vi "Calibrate sensor main.vi"() -> ()   [LabVIEW 2024]
doc: "Calibration VI"
uses:
  controls/Units.ctl
  <vilib>/Utility/miscctls.llb/LVPointTypeDef.ctl
  controls/Cal Sensor Enum.ctl
  controls/GlobalData.vi
  <userlib>/_OpenG.lib/lvdata/lvdata.llb/openg_variant.lvlib
panel:
  in  "Units Settings":T1={"Pressure"=enum."Pa", "Temperature"=enum."F", "Salinity"=enum."ppt", "Weight"=enum."ib"}
  in  "Cancel Button":bool
  in  "Weight":T2={"W C (Y-Intercept)"=0.0, "W M (Gradient)"=100.0, "Zero Weight"=FALSE, "Weight %s"=22.86994789, "W Current (mA)"=0.0, "W Save Calibration"=FALSE} {"W Current (mA)" format="%#_12g"; "Weight %s" scale=0.0..220.0}
  in  "Salinity":T3={"S C (Y-Intercept)"=0.0, "S M (Gradient)"=100.0, "Zero Salinity"=FALSE, "Salinity %s"=0.0, "S Current (mA)"=0.0, "S Save Calibration"=FALSE} {"S Current (mA)" format="%#_12g"; "Salinity %s" scale=0.0..100000.0}
  in  "Temperature":T4={"T C (Y-Intercept)"=0.0, "T M (Gradient)"=100.0, "Zero Temperature"=FALSE, "Temperature %s"=0.0, "T Current (mA)"=0.0, "T Save Calibration"=FALSE} {"T Current (mA)" format="%#_12g"; "Temperature %s" scale=0.0..100.0}
  in  "Pressure":T5={"P C (Y-Intercept)"=0.0, "P M (Gradient)"=3.0, "Zero pressure"=FALSE, "Pressure %s"=36.73931247994955, "P Current (mA)"=36.73931247994955, "P Save Calibration"=FALSE} {"P Current (mA)" format="%#_12g"; "Pressure %s" scale=0.0..60.0}
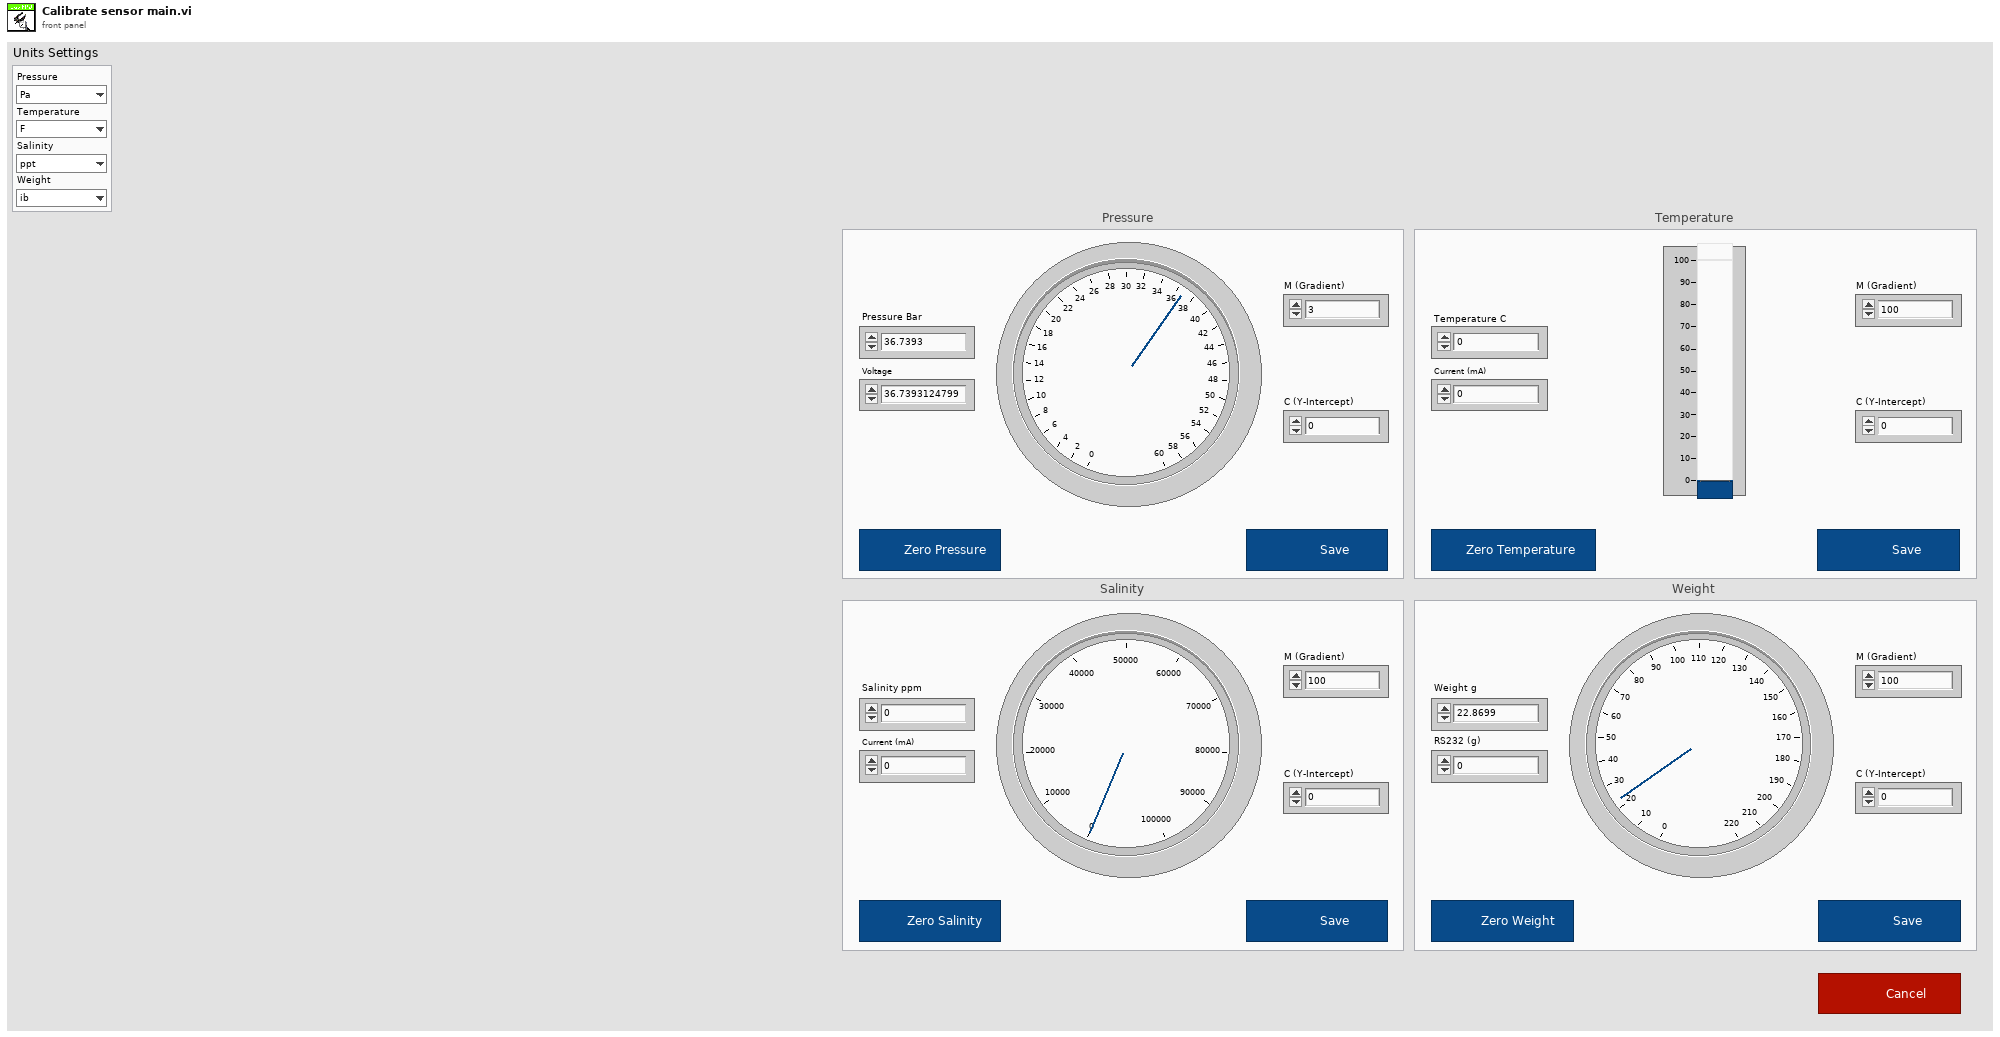
[diagram p1: front panel]
types:
  T1 = typedef "Units.ctl" = cluster{"Pressure":enum16{"PSI", "Bar", "atm", "Pa"}, "Temperature":enum16{"C", "K", "F"}, "Salinity":enum16{"ppm", "ppt", "PSU"}, "Weight":enum16{"Kg", "g", "oz", "ib"}}
  T2 = cluster{"W C (Y-Intercept)":dbl, "W M (Gradient)":dbl, "Zero Weight":bool, "Weight %s":dbl, "W Current (mA)":dbl, "W Save Calibration":bool}
  T3 = cluster{"S C (Y-Intercept)":dbl, "S M (Gradient)":dbl, "Zero Salinity":bool, "Salinity %s":dbl, "S Current (mA)":dbl, "S Save Calibration":bool}
  T4 = cluster{"T C (Y-Intercept)":dbl, "T M (Gradient)":dbl, "Zero Temperature":bool, "Temperature %s":dbl, "T Current (mA)":dbl, "T Save Calibration":bool}
  T5 = cluster{"P C (Y-Intercept)":dbl, "P M (Gradient)":dbl, "Zero pressure":bool, "Pressure %s":dbl, "P Current (mA)":dbl, "P Save Calibration":bool}
  T6 = typedef "LVPointTypeDef.ctl" = cluster{"Horizontal":i16, "Vertical":i16}
  T7 = typedef "GlobalData.ctl" = cluster{"Measurements":cluster{"Measurement Graphs":refnum<vi>, "Pressure":refnum<vi>, "Temperature":refnum<vi>, "Salinity":refnum<vi>, "Weight":refnum<vi>, "Pressure Raw":refnum<vi>, "Temperature Raw":refnum<vi>, "Salinity Raw":refnum<vi>, "Weight Raw":refnum<vi>, "Measurement Statstics":refnum<vi>, "Time Array":refnum<vi>}, "Settings":cluster{"Sampling Settings":refnum<vi>, "General Settings":refnum<vi>, "Disable Sensor Reading":refnum<vi>, "Units Settings":refnum<vi>, "Channels Settings":refnum<vi>, "Weight Port Settings":refnum<vi>}, "Calibration Data":cluster{"Pressure Cal":refnum<vi>, "Temperature Cal":refnum<vi>, "Salinity Cal":refnum<vi>, "Weight Cal":refnum<vi>}, "UI":cluster{"Generate Report":refnum<vi>}}
  T8 = cluster{"Reading Time (ms)":u64, "Graph Time ":u16}
  T9 = cluster{"C (Y-Intercept)":dbl, "M (Gradient)":dbl}
  T10 = enum32{"Invalid", "Standard", "Closed", "Hidden", "Minimized", "Maximized"}
  T11 = typedef "Cal Sensor Enum.ctl" = enum16{"All", "Pressure", "Temperature", "Salinity", "Weight"}
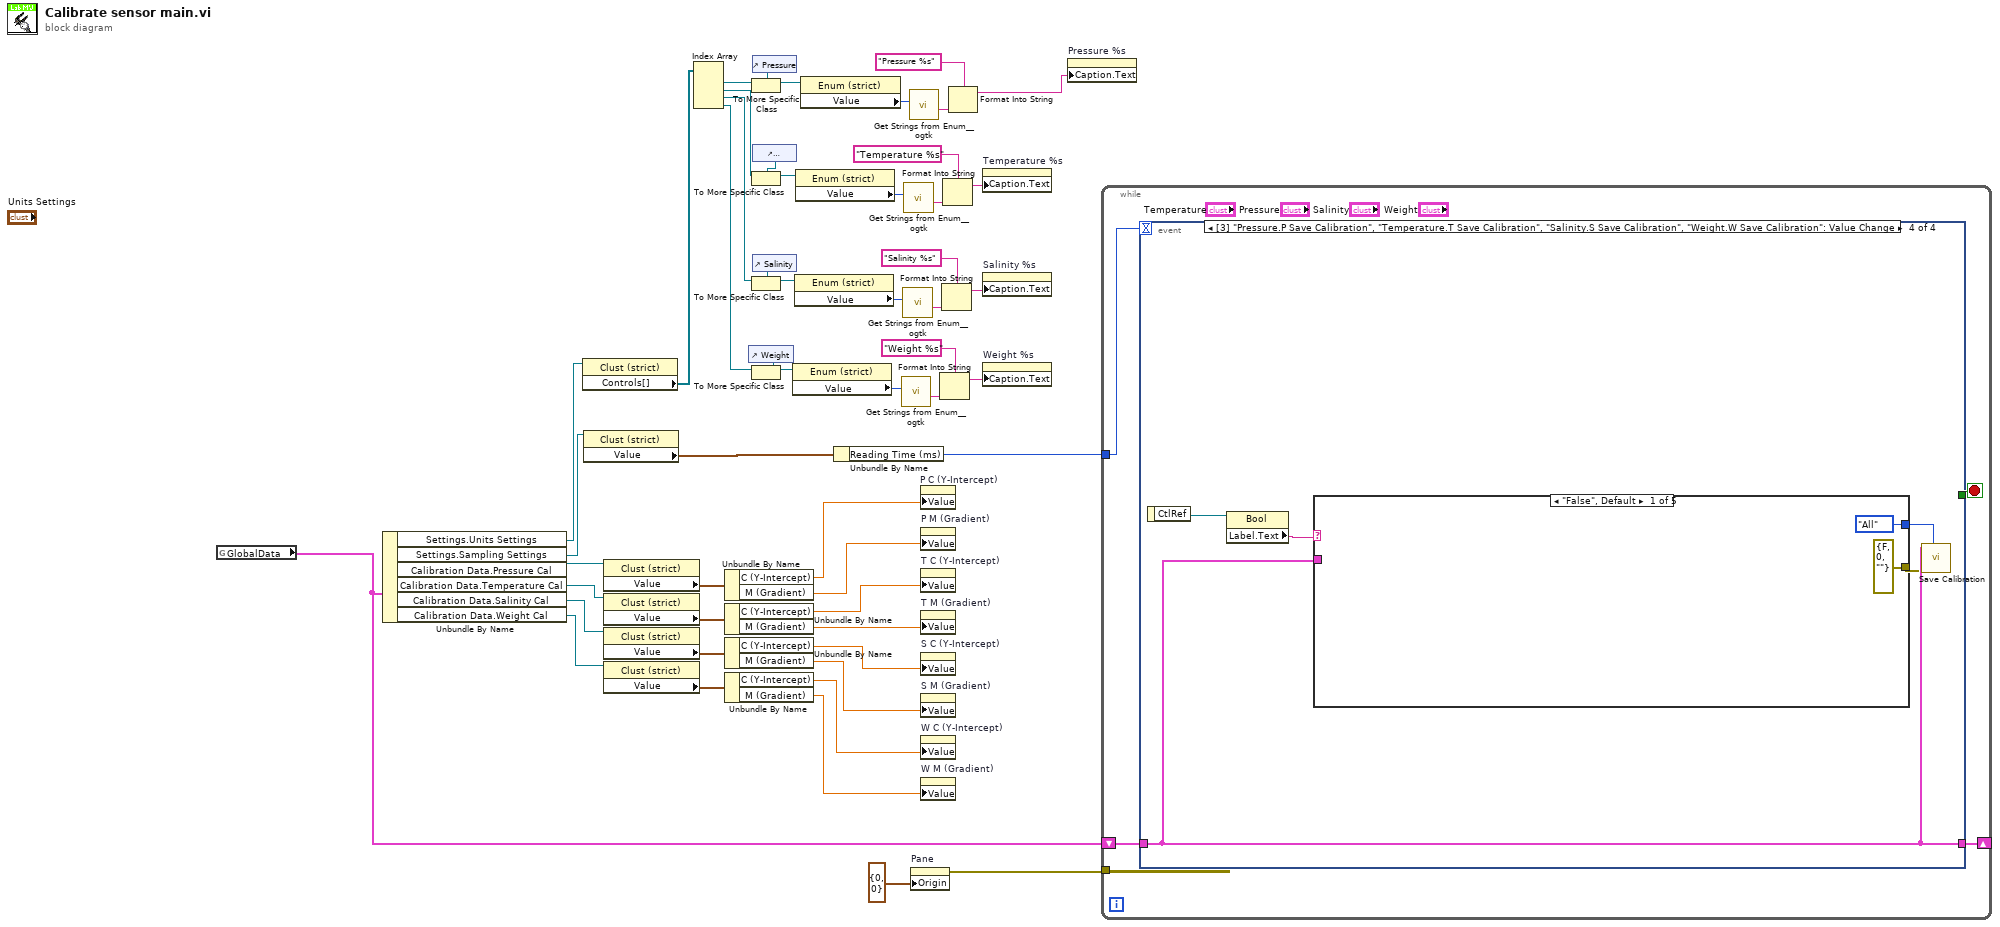
[diagram p0: block diagram]
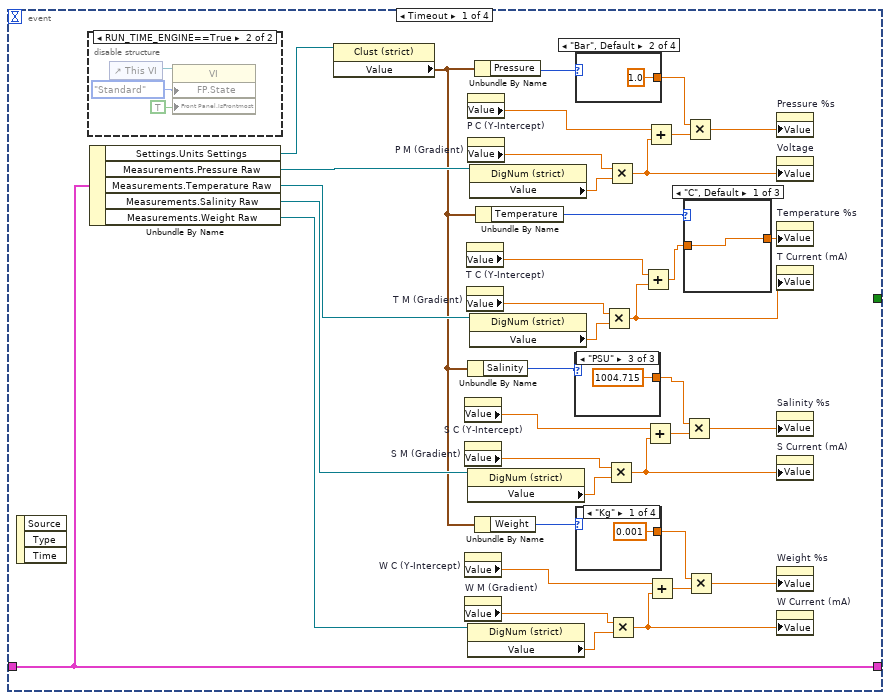
[diagram p2: hidden frame]
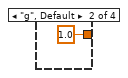
[diagram p3: hidden frame]
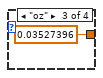
[diagram p4: hidden frame]
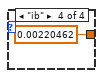
[diagram p5: hidden frame]
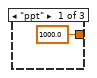
[diagram p6: hidden frame]
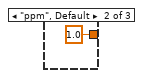
[diagram p7: hidden frame]
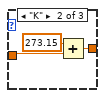
[diagram p8: hidden frame]
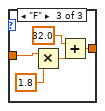
[diagram p9: hidden frame]
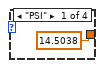
[diagram p10: hidden frame]
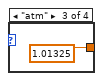
[diagram p11: hidden frame]
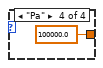
[diagram p12: hidden frame]
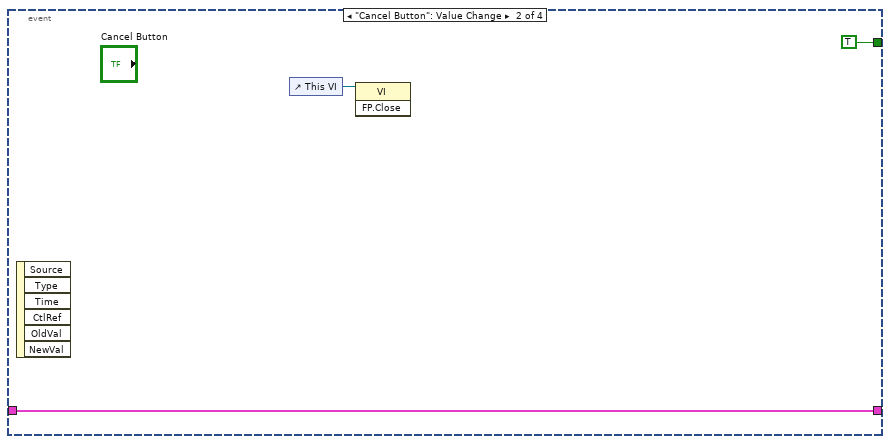
[diagram p14: hidden frame]
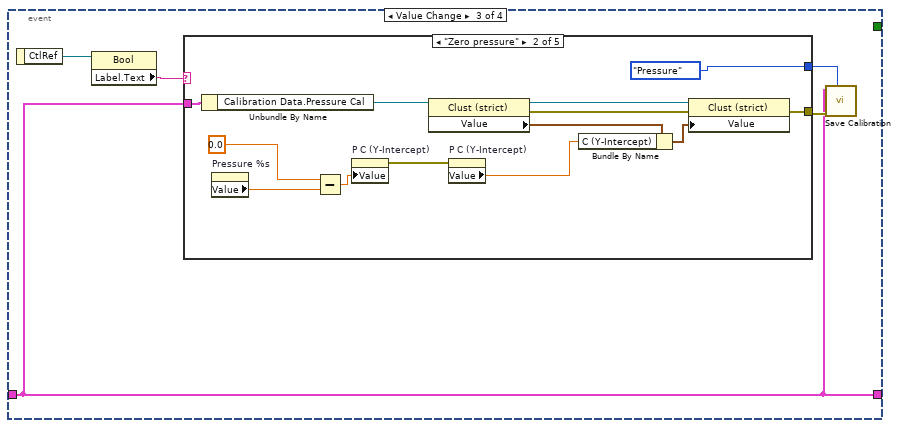
[diagram p15: hidden frame]
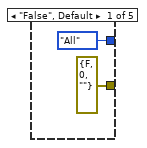
[diagram p16: hidden frame]
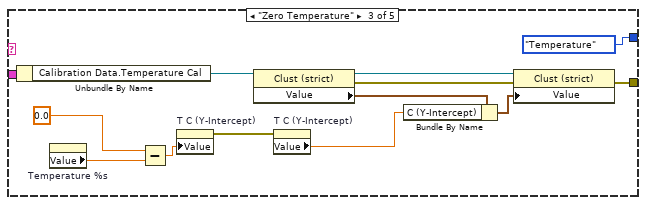
[diagram p17: hidden frame]
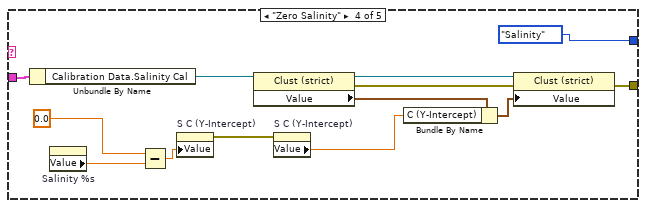
[diagram p18: hidden frame]
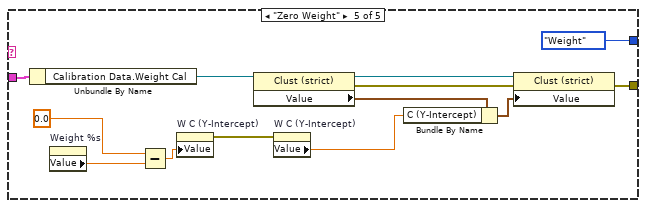
[diagram p19: hidden frame]
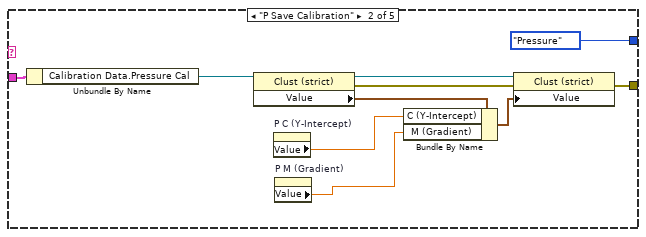
[diagram p20: hidden frame]
diagram:
  n1 = global read "GlobalData.vi" "GlobalData"() -> (w4:T7)
  n2 = Unbundle By Name(w4) -> ("Settings.Units Settings"=w3:refnum<vi>, "Settings.Sampling Settings"=w34:refnum<vi>, "Calibration Data.Pressure Cal"=w50:refnum<vi>, "Calibration Data.Temperature Cal"=w45:refnum<vi>, "Calibration Data.Salinity Cal"=w44:refnum<vi>, "Calibration Data.Weight Cal"=w43:refnum<vi>)
  n3 = property class="Clust (strict)"(reference=w3) -> ("Controls[]"=w2:refnum<vi>[])  [unwired: 1 in, 2 out]
  n4 = property class="Clust (strict)"(reference=w34) -> ("Value"=w13:T8)  [unwired: 1 in, 2 out]
  n5 = property class="Clust (strict)"(reference=w50) -> ("Value"=w49:T9)  [unwired: 1 in, 2 out]
  n6 = property class="Clust (strict)"(reference=w45) -> ("Value"=w48:T9)  [unwired: 1 in, 2 out]
  n7 = property class="Clust (strict)"(reference=w44) -> ("Value"=w46:T9)  [unwired: 1 in, 2 out]
  n8 = property class="Clust (strict)"(reference=w43) -> ("Value"=w47:T9)  [unwired: 1 in, 2 out]
  n9 = Index Array(array=w2) -> (element #1=w29:refnum<vi>, element #2=w19:refnum<vi>, element #3=w18:refnum<vi>, element #4=w17:refnum<vi>)  [unwired: 4 in]
  n10 = Unbundle By Name(w49) -> ("C (Y-Intercept)"=w42:dbl, "M (Gradient)"=w41:dbl)
  n11 = Unbundle By Name(w48) -> ("C (Y-Intercept)"=w39:dbl, "M (Gradient)"=w40:dbl)
  n12 = Unbundle By Name(w46) -> ("C (Y-Intercept)"=w38:dbl, "M (Gradient)"=w37:dbl)
  n13 = Unbundle By Name(w47) -> ("C (Y-Intercept)"=w36:dbl, "M (Gradient)"=w35:dbl)
  n14 = control-ref of="Weight"() -> (w5:refnum<vi>)
  n15 = To More Specific Class(target class=w5, reference=w17) -> (specific class reference=w20:refnum<vi>)  [unwired: 1 in, 1 out]
  n16 = control-ref of="Pressure"() -> (w8:refnum<vi>)
  n17 = To More Specific Class(target class=w8, reference=w29) -> (specific class reference=w32:refnum<vi>)  [unwired: 1 in, 1 out]
  n18 = control-ref of="Temperature"() -> (w7:refnum<vi>)
  n19 = To More Specific Class(target class=w7, reference=w19) -> (specific class reference=w26:refnum<vi>)  [unwired: 1 in, 1 out]
  n20 = control-ref of="Salinity"() -> (w6:refnum<vi>)
  n21 = To More Specific Class(target class=w6, reference=w18) -> (specific class reference=w25:refnum<vi>)  [unwired: 1 in, 1 out]
  n22 = property on="Property Node" class="Enum (strict)"(reference=w20) -> ("Value"=w21:enum16{"Kg", "g", "oz", "ib"})  [unwired: 1 in, 2 out]
  n23 = property on="Property Node" class="Enum (strict)"(reference=w25) -> ("Value"=w24:enum16{"ppm", "ppt", "PSU"})  [unwired: 1 in, 2 out]
  n24 = property on="Property Node" class="Enum (strict)"(reference=w26) -> ("Value"=w27:enum16{"C", "K", "F"})  [unwired: 1 in, 2 out]
  n25 = property on="Property Node" class="Enum (strict)"(reference=w32) -> ("Value"=w31:enum16{"PSI", "Bar", "atm", "Pa"})  [unwired: 1 in, 2 out]
  n26 = Unbundle By Name(w13) -> ("Reading Time (ms)"=w33:u64)
  n27 = call <userlib>:"Get Strings from Enum__ogtk.vi"("Enum"=w21) -> ("String Value"=w22:string)  [unwired: 7 in, 3 out]
  n28 = call <userlib>:"Get Strings from Enum__ogtk.vi"("Enum"=w24) -> ("String Value"=w23:string)  [unwired: 7 in, 3 out]
  n29 = call <userlib>:"Get Strings from Enum__ogtk.vi"("Enum"=w27) -> ("String Value"=w28:string)  [unwired: 7 in, 3 out]
  n30 = call <userlib>:"Get Strings from Enum__ogtk.vi"("Enum"=w31) -> ("String Value"=w30:string)  [unwired: 7 in, 3 out]
  n31 = property on="Pane" class="Pane"("Origin"=T6 {"Horizontal"=0, "Vertical"=0}) -> (error out=w51:errorcluster)  [unwired: 2 in, 1 out]
  n32 = property on="P C (Y-Intercept)" class="DigNum (strict)"("Value"=w42) -> ()  [unwired: 2 in, 2 out]
  n33 = property on="P M (Gradient)" class="DigNum (strict)"("Value"=w41) -> ()  [unwired: 2 in, 2 out]
  n34 = property on="T C (Y-Intercept)" class="DigNum (strict)"("Value"=w39) -> ()  [unwired: 2 in, 2 out]
  n35 = property on="T M (Gradient)" class="DigNum (strict)"("Value"=w40) -> ()  [unwired: 2 in, 2 out]
  n36 = property on="S C (Y-Intercept)" class="DigNum (strict)"("Value"=w38) -> ()  [unwired: 2 in, 2 out]
  n37 = property on="S M (Gradient)" class="DigNum (strict)"("Value"=w37) -> ()  [unwired: 2 in, 2 out]
  n38 = property on="W C (Y-Intercept)" class="DigNum (strict)"("Value"=w36) -> ()  [unwired: 2 in, 2 out]
  n39 = property on="W M (Gradient)" class="DigNum (strict)"("Value"=w35) -> ()  [unwired: 2 in, 2 out]
  n40 = Format Into String(format string="Weight %s", w22) -> (resulting string=w15:string)  [unwired: 2 in, 1 out]
  n41 = Format Into String(format string="Salinity %s", w23) -> (resulting string=w14:string)  [unwired: 2 in, 1 out]
  n42 = Format Into String(format string="Temperature %s", w28) -> (resulting string=w16:string)  [unwired: 2 in, 1 out]
  n43 = Format Into String(format string="Pressure %s", w30) -> (resulting string=w1:string)  [unwired: 2 in, 1 out]
  n44 = property on="Temperature %s" class="Slide (strict)"("Caption.Text"=w16) -> ()  [unwired: 2 in, 2 out]
  n45 = property on="Salinity %s" class="Knob (strict)"("Caption.Text"=w14) -> ()  [unwired: 2 in, 2 out]
  n46 = property on="Weight %s" class="Knob (strict)"("Caption.Text"=w15) -> ()  [unwired: 2 in, 2 out]
  n47 = property on="Pressure %s" class="Knob (strict)"("Caption.Text"=w1) -> ()  [unwired: 2 in, 2 out]
  n48 = while {
    tunnel: w51 -> [_]
    tunnel: w33 -> [w55]
    shift-right: [w53] -> _
    shift-left: w4 -> [w54]
    stop <- w56 stop-if-true
    n49 = event shown="[3] \"Pressure.P Save Calibration\", \"Temperature.T Save Calibration\", \"Salinity.S Save Calibration\", \"Weight.W Save Calibration\": Value Change" {
      selector: _ -> [_ _ _ _]
      dyn-events: _ -> [_ _ _ _]
      timeout: w55 -> [_ _ _ _]
      tunnel: [_ TRUE _ _] -> w56
      tunnel: w54 -> [w94 w118 w122 w182]
      tunnel: [w94 w118 w122 w182] -> w53
      event Timeout {
        n50 = event-data() -> ()  [unwired: 1 in, 3 out]
        n51 = disable-structure shown="RUN_TIME_ENGINE==True" {
          frame condition #0 (active) {
          }
          frame condition #1 {
            n52 = control-ref of="This VI"() -> (w117:refnum<vi>)
            n53 = property class="VI"(reference=w117, "FP.State"=T10."Standard" ("Front Panel Window:State"), "Front Panel.IsFrontmost"=TRUE ("Front Panel Window:Is Frontmost")) -> ()  [unwired: 1 in, 2 out]
          }
        }
        n54 = Unbundle By Name(w94) -> ("Settings.Units Settings"=w84:refnum<vi>, "Measurements.Pressure Raw"=w93:refnum<vi>, "Measurements.Temperature Raw"=w92:refnum<vi>, "Measurements.Salinity Raw"=w91:refnum<vi>, "Measurements.Weight Raw"=w90:refnum<vi>)
        n55 = property class="Clust (strict)"(reference=w84) -> ("Value"=w85:T1)  [unwired: 1 in, 2 out]
        n56 = property on="S C (Y-Intercept)" class="DigNum (strict)"() -> ("Value"=w75:dbl)  [unwired: 2 in, 2 out]
        n57 = property on="S M (Gradient)" class="DigNum (strict)"() -> ("Value"=w74:dbl)  [unwired: 2 in, 2 out]
        n58 = property on="W C (Y-Intercept)" class="DigNum (strict)"() -> ("Value"=w68:dbl)  [unwired: 2 in, 2 out]
        n59 = property on="W M (Gradient)" class="DigNum (strict)"() -> ("Value"=w69:dbl)  [unwired: 2 in, 2 out]
        n60 = property on="T C (Y-Intercept)" class="DigNum (strict)"() -> ("Value"=w79:dbl)  [unwired: 2 in, 2 out]
        n61 = property on="T M (Gradient)" class="DigNum (strict)"() -> ("Value"=w80:dbl)  [unwired: 2 in, 2 out]
        n62 = property on="P C (Y-Intercept)" class="DigNum (strict)"() -> ("Value"=w86:dbl)  [unwired: 2 in, 2 out]
        n63 = property on="P M (Gradient)" class="DigNum (strict)"() -> ("Value"=w87:dbl)  [unwired: 2 in, 2 out]
        n64 = Unbundle By Name(w85) -> ("Salinity"=w60:enum16{"ppm", "ppt", "PSU"})
        n65 = property class="DigNum (strict)"(reference=w91) -> ("Value"=w76:dbl)  [unwired: 1 in, 2 out]
        n66 = property class="DigNum (strict)"(reference=w90) -> ("Value"=w70:dbl)  [unwired: 1 in, 2 out]
        n67 = property class="DigNum (strict)"(reference=w93) -> ("Value"=w88:dbl)  [unwired: 1 in, 2 out]
        n68 = property class="DigNum (strict)"(reference=w92) -> ("Value"=w81:dbl)  [unwired: 1 in, 2 out]
        n69 = Unbundle By Name(w85) -> ("Pressure"=w65:enum16{"PSI", "Bar", "atm", "Pa"})
        n70 = Unbundle By Name(w85) -> ("Weight"=w58:enum16{"Kg", "g", "oz", "ib"})
        n71 = Unbundle By Name(w85) -> ("Temperature"=w63:enum16{"C", "K", "F"})
        n72 = case shown="\"PSU\"" w60 {
          tunnel: [1000.0 ("C (Y-Intercept)") 1.0 ("C (Y-Intercept)") 1004.715 ("C (Y-Intercept)")] -> w59
          frame "ppt" {
          }
          frame "ppm", Default {
          }
          frame "PSU" {
          }
        }
        n73 = case shown="\"Bar\", Default" w65 {
          tunnel: [14.5038 ("C (Y-Intercept)") 1.0 ("C (Y-Intercept)") 1.01325 ("y") 100000.0 ("C (Y-Intercept)")] -> w64
          frame "PSI" {
          }
          frame "Bar", Default {
          }
          frame "atm" {
          }
          frame "Pa" {
          }
        }
        n74 = case shown="\"Kg\"" w58 {
          tunnel: [0.001 ("C (Y-Intercept)") 1.0 ("C (Y-Intercept)") 0.03527396 ("C (Y-Intercept)") 0.00220462 ("C (Y-Intercept)")] -> w57
          frame "Kg" {
          }
          frame "g", Default {
          }
          frame "oz" {
          }
          frame "ib" {
          }
        }
        n75 = Multiply(x=w80, y=w81) -> (x*y=w78:dbl)
        n76 = Multiply(x=w74, y=w76) -> (x*y=w72:dbl)
        n77 = Multiply(x=w87, y=w88) -> (x*y=w82:dbl)
        n78 = Multiply(x=w69, y=w70) -> (x*y=w66:dbl)
        n79 = Add(x=w79, y=w78) -> (x+y=w62:dbl)
        n80 = Add(x=w75, y=w72) -> (x+y=w77:dbl)
        n81 = Add(x=w86, y=w82) -> (x+y=w89:dbl)
        n82 = Add(x=w68, y=w66) -> (x+y=w71:dbl)
        n83 = case shown="\"C\", Default" w63 {
          tunnel: [w102 w105 w110] -> w61
          tunnel: w62 -> [w102 w104 w107]
          frame "C", Default {
          }
          frame "K" {
            n84 = Add(x=273.15, y=w104) -> (x+y=w105:dbl)
          }
          frame "F" {
            n85 = Multiply(x=w107, y=1.8 ("x")) -> (x*y=w108:dbl)
            n86 = Add(x=32.0, y=w108) -> (x+y=w110:dbl)
          }
        }
        n87 = Multiply(x=w59, y=w77) -> (x*y=w73:dbl)
        n88 = Multiply(x=w64, y=w89) -> (x*y=w83:dbl)
        n89 = Multiply(x=w57, y=w71) -> (x*y=w67:dbl)
        n90 = property on="Pressure %s" class="DigNum (strict)"("Value"=w83) -> ()  [unwired: 2 in, 2 out]
        n91 = property on="Voltage" class="DigNum (strict)"("Value"=w82) -> ()  [unwired: 2 in, 2 out]
        n92 = property on="Temperature %s" class="Slide (strict)"("Value"=w61) -> ()  [unwired: 2 in, 2 out]
        n93 = property on="T Current (mA)" class="DigNum (strict)"("Value"=w78) -> ()  [unwired: 2 in, 2 out]
        n94 = property on="Salinity %s" class="Knob (strict)"("Value"=w73) -> ()  [unwired: 2 in, 2 out]
        n95 = property on="S Current (mA)" class="DigNum (strict)"("Value"=w72) -> ()  [unwired: 2 in, 2 out]
        n96 = property on="Weight %s" class="Knob (strict)"("Value"=w67) -> ()  [unwired: 2 in, 2 out]
        n97 = property on="W Current (mA)" class="DigNum (strict)"("Value"=w66) -> ()  [unwired: 2 in, 2 out]
      }
      event "Cancel Button": Value Change {
        n98 = event-data() -> ()  [unwired: 1 in, 6 out]
        n99 = control-ref of="This VI"() -> (w119:refnum<vi>)
        n100 = invoke class="VI" method="FP.Close"(reference=w119) -> ()  [unwired: 2 in, 3 out]
      }
      event "Pressure.Zero pressure", "Temperature.Zero Temperature", "Salinity.Zero Salinity", "Weight.Zero Weight": Value Change {
        n101 = event-data() -> ("CtlRef"=w125:refnum<vi>)  [unwired: 1 in]
        n102 = property class="Bool"(reference=w125) -> ("Label.Text"=w124:string)  [unwired: 1 in, 2 out]
        n103 = case shown="\"Zero pressure\"" w124 {
          tunnel: w122 -> [_ w136 w149 w162 w175]
          tunnel: [errorcluster {"status"=FALSE, "code"=0, "source"=""} ("error out") w129 w142 w155 w168] -> w123
          tunnel: [Cal_Sensor_Enum."All" ("Calibration Sensor") Cal_Sensor_Enum."Pressure" ("Calibration Sensor") Cal_Sensor_Enum."Temperature" ("Calibration Sensor") Cal_Sensor_Enum."Salinity" ("Calibration Sensor") Cal_Sensor_Enum."Weight" ("Calibration Sensor")] -> w121
          frame "False", Default {
          }
          frame "Zero pressure" {
            n104 = Unbundle By Name(w136) -> ("Calibration Data.Pressure Cal"=w135:refnum<vi>)
            n105 = property on="Pressure %s" class="Knob (strict)"() -> ("Value"=w139:dbl)  [unwired: 2 in, 2 out]
            n106 = Subtract(x=0.0, y=w139) -> (x-y=w138:dbl)
            n107 = property on="P C (Y-Intercept)" class="DigNum (strict)"("Value"=w138) -> (error out=w140:errorcluster)  [unwired: 2 in, 1 out]
            n108 = property class="Clust (strict)"(reference=w135) -> (reference out=w134:refnum<vi>, error out=w133:errorcluster, "Value"=w132:T9)  [unwired: 1 in]
            n109 = property on="P C (Y-Intercept)" class="DigNum (strict)"(error in=w140) -> ("Value"=w130:dbl)  [unwired: 1 in, 2 out]
            n110 = Bundle By Name(cluster=w132, "C (Y-Intercept)"=w130) -> (w131:T9)
            n111 = property class="Clust (strict)"(reference=w134, error in=w133, "Value"=w131) -> (error out=w129:errorcluster)  [unwired: 1 out]
          }
          frame "Zero Temperature" {
            n112 = Unbundle By Name(w149) -> ("Calibration Data.Temperature Cal"=w148:refnum<vi>)
            n113 = property on="Temperature %s" class="Slide (strict)"() -> ("Value"=w152:dbl)  [unwired: 2 in, 2 out]
            n114 = Subtract(x=0.0, y=w152) -> (x-y=w151:dbl)
            n115 = property on="T C (Y-Intercept)" class="DigNum (strict)"("Value"=w151) -> (error out=w153:errorcluster)  [unwired: 2 in, 1 out]
            n116 = property class="Clust (strict)"(reference=w148) -> (reference out=w147:refnum<vi>, error out=w146:errorcluster, "Value"=w145:T9)  [unwired: 1 in]
            n117 = property on="T C (Y-Intercept)" class="DigNum (strict)"(error in=w153) -> ("Value"=w143:dbl)  [unwired: 1 in, 2 out]
            n118 = Bundle By Name(cluster=w145, "C (Y-Intercept)"=w143) -> (w144:T9)
            n119 = property class="Clust (strict)"(reference=w147, error in=w146, "Value"=w144) -> (error out=w142:errorcluster)  [unwired: 1 out]
          }
          frame "Zero Salinity" {
            n120 = Unbundle By Name(w162) -> ("Calibration Data.Salinity Cal"=w161:refnum<vi>)
            n121 = property on="Salinity %s" class="Knob (strict)"() -> ("Value"=w165:dbl)  [unwired: 2 in, 2 out]
            n122 = Subtract(x=0.0, y=w165) -> (x-y=w164:dbl)
            n123 = property on="S C (Y-Intercept)" class="DigNum (strict)"("Value"=w164) -> (error out=w166:errorcluster)  [unwired: 2 in, 1 out]
            n124 = property class="Clust (strict)"(reference=w161) -> (reference out=w160:refnum<vi>, error out=w159:errorcluster, "Value"=w158:T9)  [unwired: 1 in]
            n125 = property on="S C (Y-Intercept)" class="DigNum (strict)"(error in=w166) -> ("Value"=w156:dbl)  [unwired: 1 in, 2 out]
            n126 = Bundle By Name(cluster=w158, "C (Y-Intercept)"=w156) -> (w157:T9)
            n127 = property class="Clust (strict)"(reference=w160, error in=w159, "Value"=w157) -> (error out=w155:errorcluster)  [unwired: 1 out]
          }
          frame "Zero Weight" {
            n128 = Unbundle By Name(w175) -> ("Calibration Data.Weight Cal"=w174:refnum<vi>)
            n129 = property on="Weight %s" class="Knob (strict)"() -> ("Value"=w178:dbl)  [unwired: 2 in, 2 out]
            n130 = Subtract(x=0.0, y=w178) -> (x-y=w177:dbl)
            n131 = property on="W C (Y-Intercept)" class="DigNum (strict)"("Value"=w177) -> (error out=w179:errorcluster)  [unwired: 2 in, 1 out]
            n132 = property class="Clust (strict)"(reference=w174) -> (reference out=w173:refnum<vi>, error out=w172:errorcluster, "Value"=w171:T9)  [unwired: 1 in]
            n133 = property on="W C (Y-Intercept)" class="DigNum (strict)"(error in=w179) -> ("Value"=w169:dbl)  [unwired: 1 in, 2 out]
            n134 = Bundle By Name(cluster=w171, "C (Y-Intercept)"=w169) -> (w170:T9)
            n135 = property class="Clust (strict)"(reference=w173, error in=w172, "Value"=w170) -> (error out=w168:errorcluster)  [unwired: 1 out]
          }
        }
        n136 = call "Save Calibration.vi"("Calibration Sensor"=w121, "error in (no error)"=w123, "GlobalData"=w122) -> ()  [unwired: 8 in, 1 out]
      }
      event "Pressure.P Save Calibration", "Temperature.T Save Calibration", "Salinity.S Save Calibration", "Weight.W Save Calibration": Value Change {
        n137 = event-data() -> ("CtlRef"=w184:refnum<vi>)  [unwired: 1 in]
        n138 = property class="Bool"(reference=w184) -> ("Label.Text"=w183:string)  [unwired: 1 in, 2 out]
        n139 = case shown="\"False\", Default" w183 {
          tunnel: w182 -> [_ w196 w206 w216 w226]
          tunnel: [errorcluster {"status"=FALSE, "code"=0, "source"=""} ("error out") w189 w199 w209 w219] -> w181
          tunnel: [Cal_Sensor_Enum."All" ("Calibration Sensor") Cal_Sensor_Enum."Pressure" ("Calibration Sensor") Cal_Sensor_Enum."Temperature" ("Calibration Sensor") Cal_Sensor_Enum."Salinity" ("Calibration Sensor") Cal_Sensor_Enum."Weight" ("Calibration Sensor")] -> w180
          frame "False", Default {
          }
          frame "P Save Calibration" {
            n140 = Unbundle By Name(w196) -> ("Calibration Data.Pressure Cal"=w195:refnum<vi>)
            n141 = property class="Clust (strict)"(reference=w195) -> (reference out=w194:refnum<vi>, error out=w193:errorcluster, "Value"=w192:T9)  [unwired: 1 in]
            n142 = property on="P C (Y-Intercept)" class="DigNum (strict)"() -> ("Value"=w190:dbl)  [unwired: 2 in, 2 out]
            n143 = property on="P M (Gradient)" class="DigNum (strict)"() -> ("Value"=w187:dbl)  [unwired: 2 in, 2 out]
            n144 = Bundle By Name(cluster=w192, "C (Y-Intercept)"=w190, "M (Gradient)"=w187) -> (w191:T9)
            n145 = property class="Clust (strict)"(reference=w194, error in=w193, "Value"=w191) -> (error out=w189:errorcluster)  [unwired: 1 out]
          }
          frame "T Save Calibration" {
            n146 = Unbundle By Name(w206) -> ("Calibration Data.Temperature Cal"=w205:refnum<vi>)
            n147 = property class="Clust (strict)"(reference=w205) -> (reference out=w204:refnum<vi>, error out=w203:errorcluster, "Value"=w202:T9)  [unwired: 1 in]
            n148 = property on="T C (Y-Intercept)" class="DigNum (strict)"() -> ("Value"=w200:dbl)  [unwired: 2 in, 2 out]
            n149 = property on="T M (Gradient)" class="DigNum (strict)"() -> ("Value"=w197:dbl)  [unwired: 2 in, 2 out]
            n150 = Bundle By Name(cluster=w202, "C (Y-Intercept)"=w200, "M (Gradient)"=w197) -> (w201:T9)
            n151 = property class="Clust (strict)"(reference=w204, error in=w203, "Value"=w201) -> (error out=w199:errorcluster)  [unwired: 1 out]
          }
          frame "S Save Calibration" {
            n152 = Unbundle By Name(w216) -> ("Calibration Data.Salinity Cal"=w215:refnum<vi>)
            n153 = property class="Clust (strict)"(reference=w215) -> (reference out=w214:refnum<vi>, error out=w213:errorcluster, "Value"=w212:T9)  [unwired: 1 in]
            n154 = property on="S M (Gradient)" class="DigNum (strict)"() -> ("Value"=w207:dbl)  [unwired: 2 in, 2 out]
            n155 = property on="S C (Y-Intercept)" class="DigNum (strict)"() -> ("Value"=w210:dbl)  [unwired: 2 in, 2 out]
            n156 = Bundle By Name(cluster=w212, "C (Y-Intercept)"=w210, "M (Gradient)"=w207) -> (w211:T9)
            n157 = property class="Clust (strict)"(reference=w214, error in=w213, "Value"=w211) -> (error out=w209:errorcluster)  [unwired: 1 out]
          }
          frame "W Save Calibration" {
            n158 = Unbundle By Name(w226) -> ("Calibration Data.Weight Cal"=w225:refnum<vi>)
            n159 = property class="Clust (strict)"(reference=w225) -> (reference out=w224:refnum<vi>, error out=w223:errorcluster, "Value"=w222:T9)  [unwired: 1 in]
            n160 = property on="W M (Gradient)" class="DigNum (strict)"() -> ("Value"=w217:dbl)  [unwired: 2 in, 2 out]
            n161 = property on="W C (Y-Intercept)" class="DigNum (strict)"() -> ("Value"=w220:dbl)  [unwired: 2 in, 2 out]
            n162 = Bundle By Name(cluster=w222, "C (Y-Intercept)"=w220, "M (Gradient)"=w217) -> (w221:T9)
            n163 = property class="Clust (strict)"(reference=w224, error in=w223, "Value"=w221) -> (error out=w219:errorcluster)  [unwired: 1 out]
          }
        }
        n164 = call "Save Calibration.vi"("Calibration Sensor"=w180, "error in (no error)"=w181, "GlobalData"=w182) -> ()  [unwired: 8 in, 1 out]
      }
    }
  }
